vi "ResetFrontPanel.vi"(8 "Error In":errorcluster, 11 "VI Path":path) -> (0 "Error Out":errorcluster)   [LabVIEW 2012, in "LV-Utilities.lvlib"]
uses:
  LV-Utilities.lvlib
  <vilib>/Utility/miscctls.llb/LVPointTypeDef.ctl
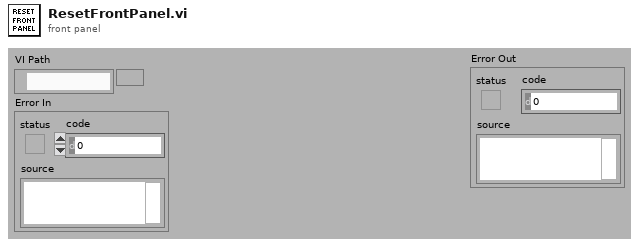
[diagram p1: front panel]
types:
  T1 = typedef "LVPointTypeDef.ctl" = cluster{"Horizontal":i16, "Vertical":i16}
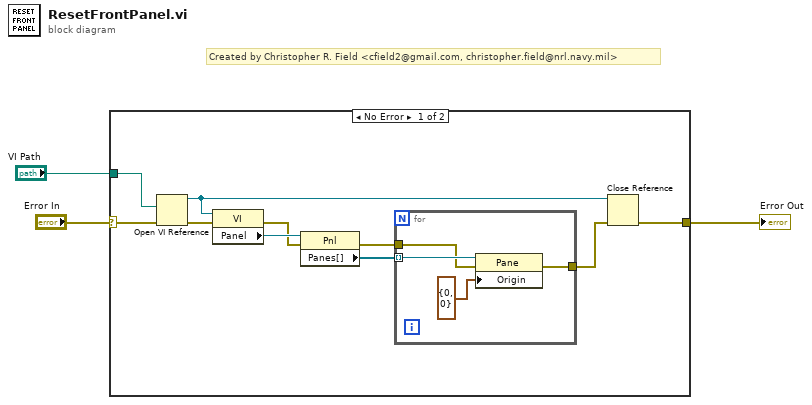
[diagram p0: block diagram]
diagram:
  # "Created by Christopher R. Field <cfield2@gmail.com, christopher.field@nrl.navy.mil>"
  n1 = case shown="No Error" "Error In" {
    selector: "Error In" -> [w4 w18]
    tunnel: "VI Path" -> [w13 _]
    tunnel: [w5 w18] -> w2
    frame No Error {
      n2 = Open VI Reference(vi path=w13, error in (no error)=w4) -> (vi reference=w6:refnum<vi>, error out=w12:errorcluster)  [unwired: 4 in]
      n3 = property class="VI"(reference=w6, error in=w12) -> (error out=w10:errorcluster, "Panel"=w11:refnum<vi>)  [unwired: 1 out]
      n4 = property class="Pnl"(reference=w11, error in=w10) -> (error out=w8:errorcluster, "Panes[]"=w9:refnum<vi>[])  [unwired: 1 out]
      n5 = for {
        tunnel: w9 -> [w17] mode=indexing
        tunnel: w8 -> [w15]
        tunnel: [w14] -> w7
        n6 = property class="Pane"(reference=w17, error in=w15, "Origin"=T1 {"Horizontal"=0, "Vertical"=0}) -> (error out=w14:errorcluster)  [unwired: 1 out]
      }
      n7 = Close Reference(reference=w6, error in (no error)=w7) -> (error out=w5:errorcluster)
    }
    frame Error {
    }
  }
  "Error Out" <- w2
